vi "Fluke Multimeter Control Panel (No Objects).vi"() -> (0 "error out":errorcluster)   [LabVIEW 2009]
doc: "(Dynamic) A user-level application that simulates the physical front panel of the Instrument. Provide the user with buttons to manually control features of the instrument, and provide indicators of its current state."
uses:
  Fluke 8840/Fluke 8840.lvlib
panel:
  in  "VISA Resource Name":refnum<visa-resource-name>="GPIB0::2::INSTR"
  in  "error in (no error)":errorcluster
  out "AutoRange":bool
  out "unit":string
  in  "Reset":bool
  in  "Read Current Value":bool
  out "Value":dbl
  in  "Set":bool
  in  "Read to Control":bool
  in  "Read":bool
  in  "trigger mode set":u16(ring) items=["internal - continuous trigger", "external - rear panel trigger with delay", "external - bus trigger with delay", "external - rear panel trigger", "external - bus trigger"]
  in  "rate set":u16(ring) items=["slow", "medium", "fast"]
  in  "range set":u16(ring)=6 items=["autorange", "200mV, 200 ohms", "2V, 2 kohms", "20V, 20 kohms", "200V, 200 kohms", "1000Vdc, 700 Vac, 2 Mohms", "20 Mohms"]
  in  "function set":u16(ring) items=["volts DC", "volts AC", "2-wire k.ohms", "4-wire k.ohms", "mA DC", "mA AC"]
  out "trigger mode":u16(ring) items=["internal - continuous trigger", "external - rear panel trigger with delay", "external - bus trigger with delay", "external - rear panel trigger", "external - bus trigger"]
  out "rate":u16(ring) items=["slow", "medium", "fast"]
  out "range":u16(ring)=6 items=["autorange", "200mV, 200 ohms", "2V, 2 kohms", "20V, 20 kohms", "200V, 200 kohms", "1000Vdc, 700 Vac, 2 Mohms", "20 Mohms"]
  out "function":u16(ring) items=["volts DC", "volts AC", "2-wire k.ohms", "4-wire k.ohms", "mA DC", "mA AC"]
  in  "stop":bool
  in  "Copy actual to set":bool
  in  "Populate fields with member data":bool
  # "Note: can't set trigger mode yet. Apparently need to create driver for the Y1 command"
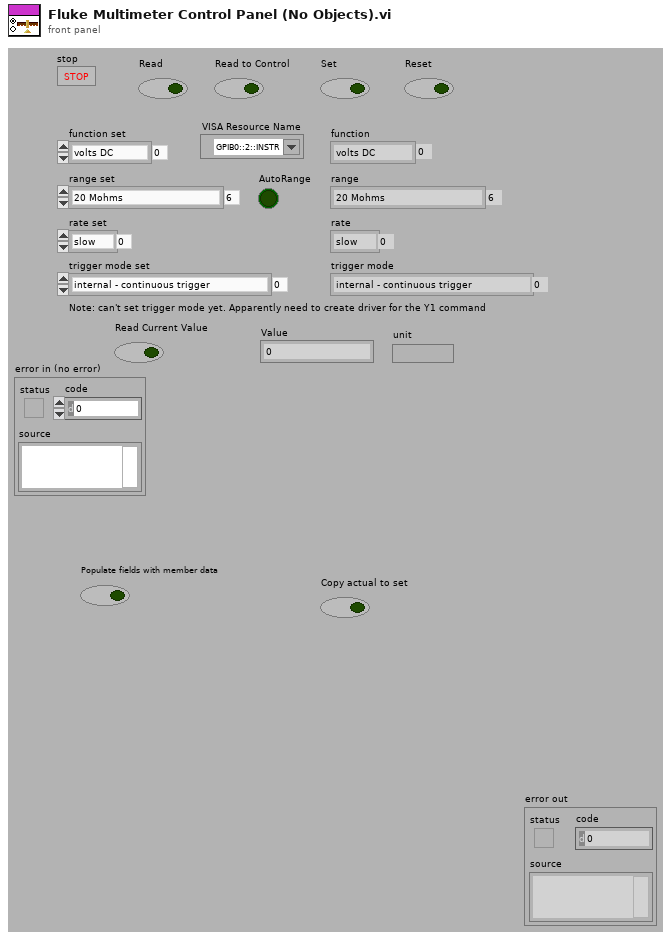
[diagram p1: front panel]
types:
  T1 = cluster{"function (0:volts DC)":u16, "range (0:auto)":u16, "rate (0:slow)":u16, "trigger mode (0:internal)":u16, "Autorange":bool}
  T2 = cluster{"function (0:volts DC)":i16, "range (0:auto)":i16, "rate (0:slow)":i16, "trigger mode (0:internal":i16, "Autorange":bool}
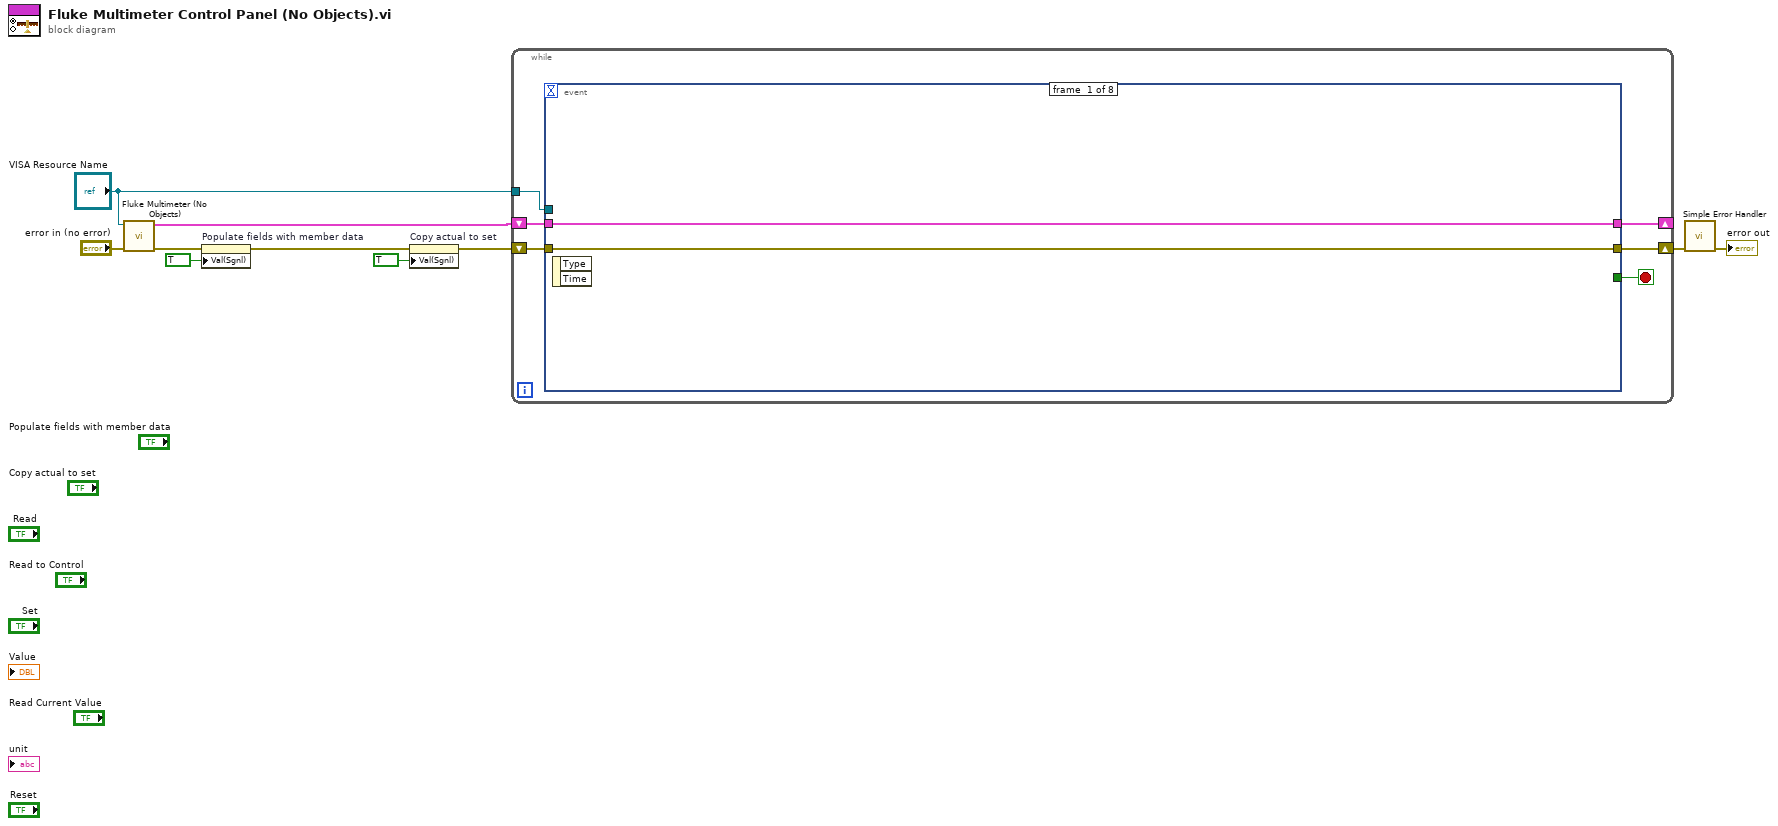
[diagram p0: block diagram]
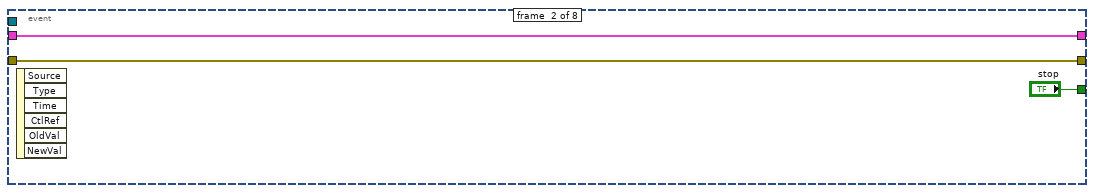
[diagram p2: hidden frame]
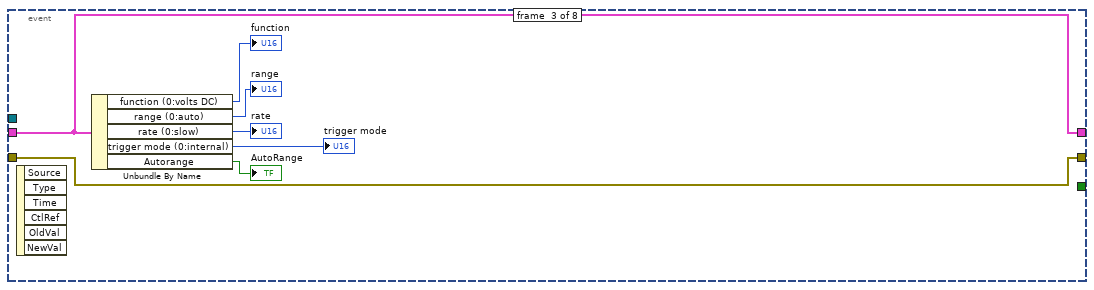
[diagram p3: hidden frame]
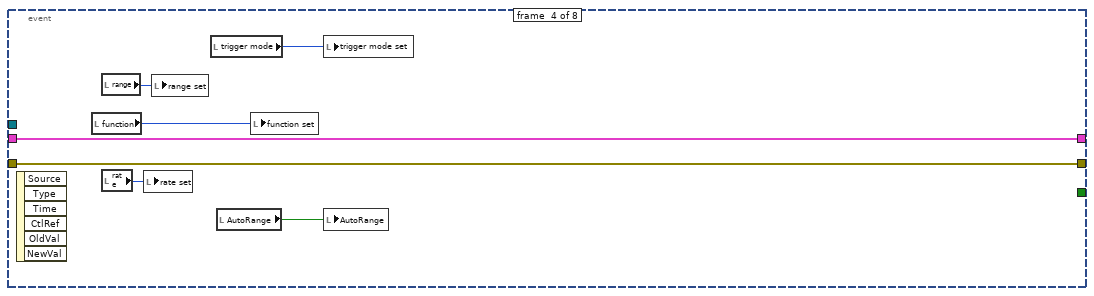
[diagram p4: hidden frame]
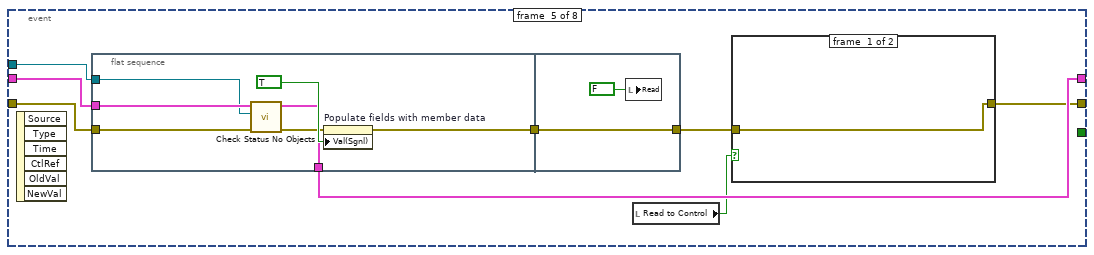
[diagram p5: hidden frame]
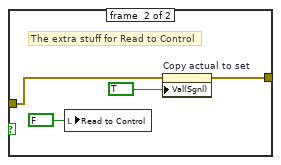
[diagram p6: hidden frame]
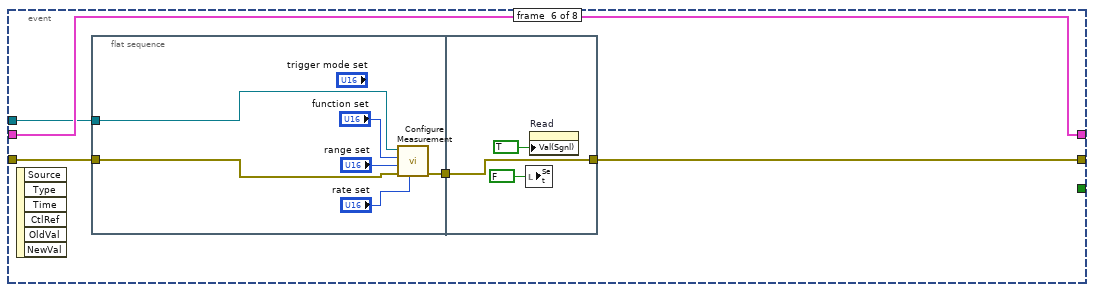
[diagram p7: hidden frame]
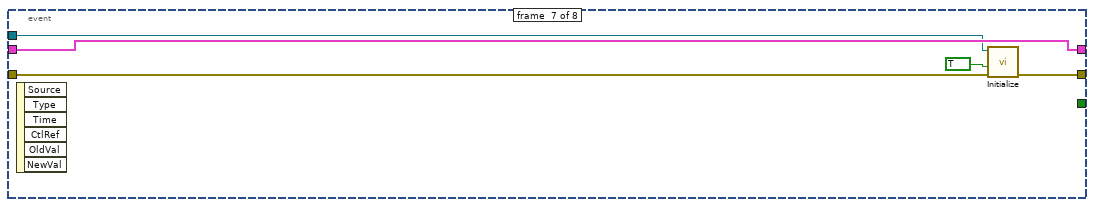
[diagram p8: hidden frame]
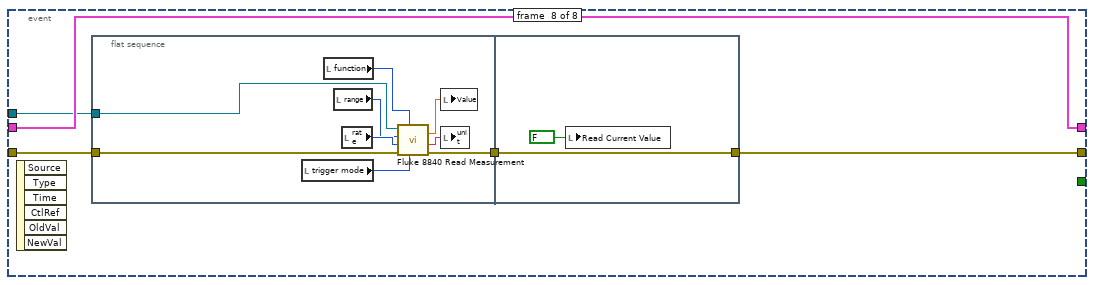
[diagram p9: hidden frame]
diagram:
  n1 = call "Fluke Multimeter (No Objects).vi"("error in (no error)"="error in (no error)", "VISA Resource Name"="VISA Resource Name") -> ("error out"=w3:errorcluster, "Fluke Multimeter out"=w2:T1)  [unwired: 8 in]
  n2 = property on="Populate fields with member data" class="Bool (strict)"(error in=w3, "Val(Sgnl)"=TRUE ("Value (Signaling)")) -> (error out=w10:errorcluster)  [unwired: 1 in, 1 out]
  n3 = property on="Copy actual to set" class="Bool (strict)"(error in=w10, "Val(Sgnl)"=TRUE ("Value (Signaling)")) -> (error out=w9:errorcluster)  [unwired: 1 in, 1 out]
  n4 = while {
    shift-right: [w13] -> _
    shift-left: w2 -> [w12]
    shift-right: [w15] -> w6
    shift-left: w9 -> [w14]
    tunnel: "VISA Resource Name" -> [w11]
    stop <- w16 stop-if-true
    n5 = event shown="[4] \"Read\", \"Read to Control\": Value Change" {
      selector: _ -> [_ _ _ _ _ _ _ _]
      dyn-events: _ -> [_ _ _ _ _ _ _ _]
      timeout: _ -> [_ _ _ _ _ _ _ _]
      tunnel: [_ "stop" _ _ _ _ _ _] -> w16
      tunnel: [w17 w20 w23 w30 w37 w61 w73 w81] -> w15
      tunnel: w14 -> [w17 w20 w23 w30 w43 w62 w74 w80]
      tunnel: [w18 w19 w24 w31 w41 w59 w75 w79] -> w13
      tunnel: w12 -> [w18 w19 w24 w31 w42 w59 w75 w79]
      tunnel: w11 -> [_ _ _ _ w36 w58 w72 w77]
      event #0 {
        n6 = event-data() -> ()  [unwired: 3 out]
      }
      event #1 {
        n7 = event-data() -> ()  [unwired: 7 out]
      }
      event #2 {
        n8 = event-data() -> ()  [unwired: 7 out]
        n9 = Unbundle By Name(w24) -> ("function (0:volts DC)"=→"function":u16, "range (0:auto)"=→"range":u16, "rate (0:slow)"=→"rate":u16, "trigger mode (0:internal)"=→"trigger mode":u16, "Autorange"=→"AutoRange":bool)
      }
      event #3 {
        n10 = event-data() -> ()  [unwired: 7 out]
        n11 = local read "function"() -> (w35:u16)
        n12 = local read "range"() -> (w34:u16)
        n13 = local read "rate"() -> (w33:u16)
        n14 = local write "rate set"(w33) -> ()
        n15 = local write "range set"(w34) -> ()
        n16 = local read "trigger mode"() -> (w32:u16)
        n17 = local read "AutoRange"() -> (w29:bool)
        n18 = local write "function set"(w35) -> ()
        n19 = local write "trigger mode set"(w32) -> ()
        n20 = local write "AutoRange"(w29) -> ()
      }
      event #4 {
        n21 = event-data() -> ()  [unwired: 7 out]
        n22 = flat-sequence {
          tunnel: w43 -> [w52]
          tunnel: w42 -> [w51]
          tunnel: [w50] -> w41
          tunnel: [w54] -> w38
          tunnel: w36 -> [w49]
          tunnel: [w56] -> w39
          tunnel: w38 -> [w56]
          frame #0 {
            n23 = call "Check Status No Objects.vi"("error in (no error)"=w52, "VISA Resource Name"=w49, "input cluster"=w51) -> ("error out"=w53:errorcluster, "output cluster"=w50:T2)  [unwired: 5 in, 2 out]
            n24 = property on="Populate fields with member data" class="Bool (strict)"(error in=w53, "Val(Sgnl)"=TRUE ("Value (Signaling)")) -> (error out=w54:errorcluster)  [unwired: 1 in, 1 out]
          }
          frame #1 {
            n25 = local write "Read"(FALSE ("Read")) -> ()
          }
        }
        n26 = local read "Read to Control"() -> (w40:bool)
        n27 = case shown="True" w40 {
          tunnel: w39 -> [w44 w46]
          tunnel: [w44 w45] -> w37
          frame #0 {
          }
          frame #1 {
            # "The extra stuff for Read to Control"
            n28 = local write "Read to Control"(FALSE ("Read to Control")) -> ()
            n29 = property on="Copy actual to set" class="Bool (strict)"(error in=w46, "Val(Sgnl)"=TRUE ("Value (Signaling)")) -> (error out=w45:errorcluster)  [unwired: 1 in, 1 out]
          }
        }
      }
      event #5 {
        n30 = event-data() -> ()  [unwired: 7 out]
        n31 = flat-sequence {
          tunnel: w62 -> [w64]
          tunnel: [w65] -> w60
          tunnel: w58 -> [w63]
          tunnel: [w71] -> w61
          tunnel: w60 -> [w71]
          frame #0 {
            n32 = call "Configure Measurement.vi"("rate (0:slow)"="rate set", "error in (no error)"=w64, "range (0:auto)"="range set", "function (0:volts DC)"="function set", "VISA resource name"=w63) -> ("error out"=w65:errorcluster)  [unwired: 6 out]
          }
          frame #1 {
            n33 = local write "Set"(FALSE ("Set")) -> ()
            n34 = property on="Read" class="Bool (strict)"("Val(Sgnl)"=TRUE ("Value (Signaling)")) -> ()  [unwired: 2 in, 2 out]
          }
        }
      }
      event #6 {
        n35 = event-data() -> ()  [unwired: 7 out]
        n36 = call "Initialize.vi"("error in (no error)"=w74, "reset (T:yes)"=TRUE, "VISA resource name"=w72) -> ("error out"=w73:errorcluster)  [unwired: 8 out]
      }
      event #7 {
        n37 = event-data() -> ()  [unwired: 7 out]
        n38 = flat-sequence {
          tunnel: w80 -> [w83]
          tunnel: [w84] -> w78
          tunnel: w77 -> [w82]
          tunnel: [w92] -> w81
          tunnel: w78 -> [w92]
          frame #0 {
            n39 = local read "trigger mode"() -> (w90:u16)
            n40 = local read "function"() -> (w87:u16)
            n41 = local read "range"() -> (w88:u16)
            n42 = local read "rate"() -> (w89:u16)
            n43 = call "Fluke 8840 Read Measurement.vi"("trigger mode (0:internal)"=w90, "function (0:volts DC)"=w87, "error in (no error)"=w83, "rate (0:slow)"=w89, "range (0:auto)"=w88, "VISA resource name"=w82) -> ("error out"=w84:errorcluster, "unit"=w85:string, "measurement"=w86:dbl)  [unwired: 3 out]
            n44 = local write "Value"(w86) -> ()
            n45 = local write "unit"(w85) -> ()
          }
          frame #1 {
            n46 = local write "Read Current Value"(FALSE ("Read Current Value")) -> ()
          }
        }
      }
    }
  }
  n47 = call <vilib>:"Simple Error Handler.vi"("error in (no error)"=w6) -> ("error out"=→"error out":errorcluster)  [unwired: 1 in, 7 out]
